vi "StartTestSuite_AfterStartTest_ReturnsError.vi"() -> (0 "error out":errorcluster)   [LabVIEW 2019, in "ResultTreeListenerTest.lvlib"]
uses:
  ResultTreeListenerTest.lvlib
  Support/FakeTestCase/FakeTestCase.lvclass
  C:/Users/de200256/Code/LVUnit/TestCase/TestCase/TestCase.lvclass
  Support/FakeTestSuite/FakeTestSuite.lvclass
  C:/Users/de200256/Code/LVUnit/TestSuite/TestSuite.lvclass
  ResultTreeListener/ResultTreeListener.lvclass
  ResultTree/ResultTree.lvclass
  Assertion/Assertion.lvlib
panel:
  in  "Tree":string(tree)
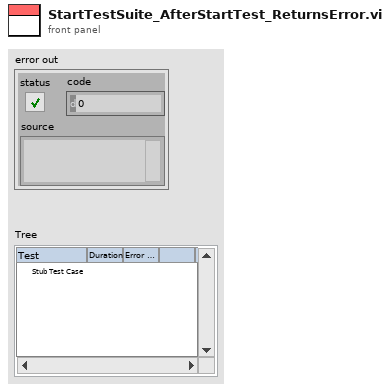
[diagram p1: front panel]
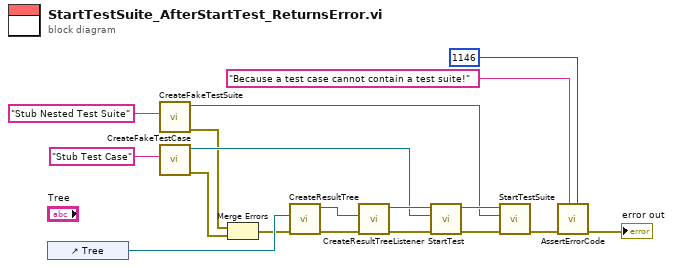
[diagram p0: block diagram]
diagram:
  n1 = control-ref of="Tree"() -> (w11:refnum<vi>)
  n2 = call "CreateFakeTestSuite.vi"("Name"="Stub Nested Test Suite") -> ("error out"=w5:errorcluster, "FakeTestSuite out"=w7:refnum<class "FakeTestSuite.lvclass">)  [unwired: 9 in]
  n3 = call "CreateFakeTestCase.vi"("Name"="Stub Test Case") -> ("error out"=w4:errorcluster, "FakeTestCase out"=w13:refnum<class "FakeTestCase.lvclass">)  [unwired: 9 in]
  n4 = Merge Errors(w5, w4) -> (w6:errorcluster)
  n5 = call "CreateResultTree.vi"("error in (no error)"=w6, "Tree Refnum"=w11) -> ("error out"=w18:errorcluster, "ResultTree out"=w17:refnum<class "ResultTree.lvclass">)  [unwired: 8 in]
  n6 = call "CreateResultTreeListener.vi"("error in (no error)"=w18, "ResultTree"=w17) -> ("error out"=w16:errorcluster, "ResultTreeListener out"=w14:refnum<class "ResultTreeListener.lvclass">)  [unwired: 8 in]
  n7 = call-dynamic "StartTest.vi"("error in (no error)"=w16, "TestCase"=w13, "ResultTreeListener in"=w14) -> ("error out"=w9:errorcluster, "ResultTreeListener out"=w8:refnum<class "ResultTreeListener.lvclass">)  [unwired: 7 in]
  n8 = call-dynamic "StartTestSuite.vi"("error in (no error)"=w9, "TestSuite"=w7, "ResultTreeListener in"=w8) -> ("error out"=w3:errorcluster)  [unwired: 7 in, 1 out]
  n9 = call "AssertErrorCode.vi"("Expected"=1146, "Message (\"\")"="Because a test case cannot contain a test suite!" ("Message (\"\")"), "error in (no error)"=w3) -> ("error out"=→"error out":errorcluster)  [unwired: 8 in]
